vi "Renderizado.vi"() -> ()   [LabVIEW 2016]
uses:
  <vilib>/picture/3D Picture Control/Object/Create Object (drawable).vi
  <vilib>/picture/3D Picture Control/Helpers/Apply Texture (no reference).vi
  <vilib>/picture/3D Picture Control/NI_3D Picture Control.lvlib
panel:
  in  "angle":sgl(knob) scale=0.0..180.0
  in  "Stop Button":bool
  in  "Path":path
  in  "Enum":enum16{"Esfera", "Cubo", "Cilindro", "Cono"}(ring)
  out "3D Picture":refnum<vi>(3d-picture)
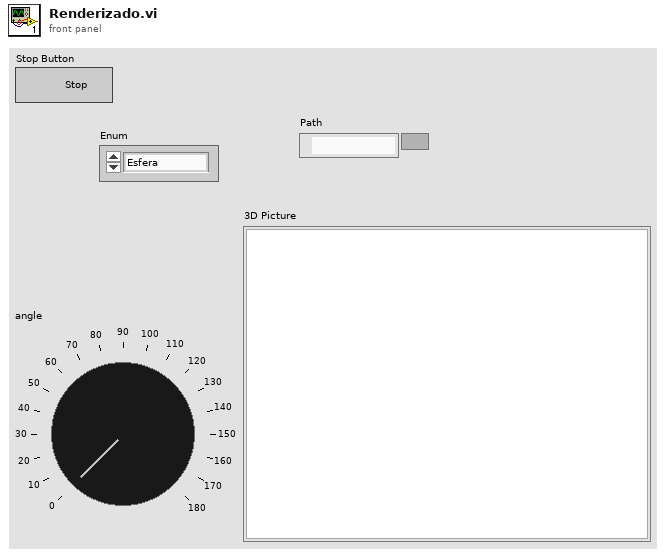
[diagram p1: front panel]
types:
  T1 = cluster{"Red":sgl, "Green":sgl, "Blue":sgl, "Alpha":sgl}
  T2 = typedef "imagedata.ctl" = cluster{"image type":i32, "image depth":i32, "image":u8[], "mask":u8[], "colors":u32[], "Rectangle":cluster{"left":i16, "top":i16, "right":i16, "bottom":i16}}
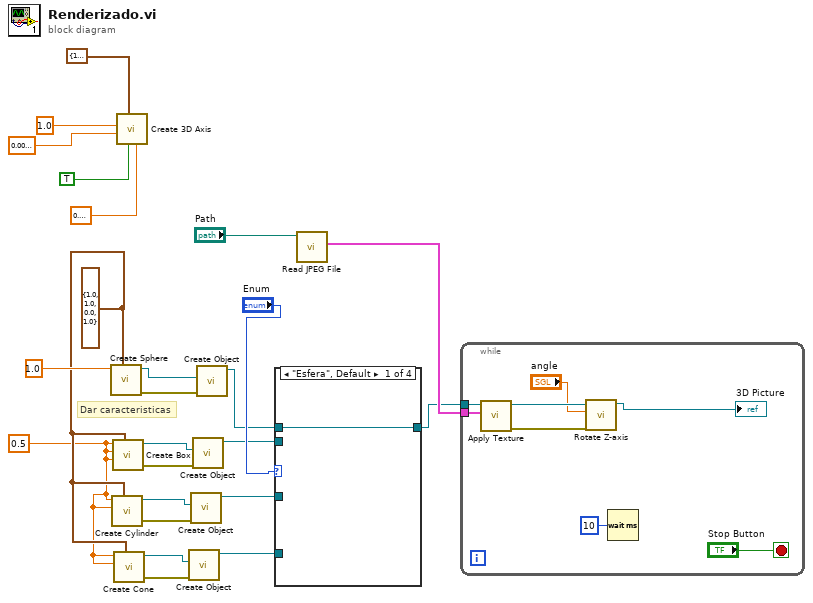
[diagram p0: block diagram]
diagram:
  w9 = sgl 0.5 ("Length X")
  w16 = T1 {"Red"=1.0, "Green"=1.0, "Blue"=0.0, "Alpha"=1.0} ("Color")
  # "Dar caracteristicas"
  n1 = call <vilib>:"Create Sphere.vi"("Color"=w16, "Radius"=sgl 1.0) -> ("error out"=w18:errorcluster, "New Sphere Refnum"=w17:refnum<vi>)  [unwired: 8 in]
  n2 = call <vilib>:"Create Cylinder.vi"("Color"=w16, "Radius"=w9, "Height"=w9) -> ("error out"=w13:errorcluster, "New Cylinder Refnum"=w12:refnum<vi>)  [unwired: 7 in]
  n3 = call <vilib>:"Create Box.vi"("Color"=w16, "Length Z"=w9, "Length Y"=w9, "Length X"=w9) -> ("error out"=w11:errorcluster, "New Box Refnum"=w10:refnum<vi>)  [unwired: 6 in]
  n4 = call <vilib>:"Create Cone.vi"("Color"=w16, "Radius"=w9, "Height"=w9) -> ("error out"=w15:errorcluster, "New Cone Refnum"=w14:refnum<vi>)  [unwired: 7 in]
  n5 = call <vilib>:"Create 3D Axis.vi"("Character Size"=sgl 0.1, "Axis label?"=TRUE, "Color"=T1 {"Red"=1.0, "Green"=0.0, "Blue"=0.0, "Alpha"=1.0}, "Radius"=sgl 0.01, "Length"=sgl 1.0) -> ()  [unwired: 5 in, 2 out]
  n6 = call-poly <vilib>:"Create Object.vi"("error in (no error)"=w15, "Geometry"=w14) -> ("Scene:New Object"=w4:refnum<vi>)  [unwired: 8 in, 1 out]
  n7 = call-poly <vilib>:"Create Object.vi"("error in (no error)"=w13, "Geometry"=w12) -> ("Scene:New Object"=w5:refnum<vi>)  [unwired: 8 in, 1 out]
  n8 = call-poly <vilib>:"Create Object.vi"("error in (no error)"=w11, "Geometry"=w10) -> ("Scene:New Object"=w6:refnum<vi>)  [unwired: 8 in, 1 out]
  n9 = call-poly <vilib>:"Create Object.vi"("error in (no error)"=w18, "Geometry"=w17) -> ("Scene:New Object"=w7:refnum<vi>)  [unwired: 8 in, 1 out]
  n10 = case shown="\"Esfera\", Default" "Enum" {
    tunnel: w7 -> [w25 _ _ _]
    tunnel: [w25 w26 w27 w28] -> w1
    tunnel: w6 -> [_ w26 _ _]
    tunnel: w5 -> [_ _ w27 _]
    tunnel: w4 -> [_ _ _ w28]
    frame "Esfera", Default {
    }
    frame "Cubo" {
    }
    frame "Cilindro" {
    }
    frame "Cono" {
    }
  }
  n11 = call <vilib>:"Read JPEG File.vi"("path to JPEG file"="Path") -> ("image data"=w2:T2)  [unwired: 8 in, 2 out]
  n12 = while {
    tunnel: w2 -> [w36]
    tunnel: w1 -> [w35]
    stop <- "Stop Button" stop-if-true
    n13 = call-poly <vilib>:"Apply Texture.vi"("Image Data"=w36, "Scene Object In"=w35) -> ("error out"=w31:errorcluster, "Scene Object Out"=w32:refnum<vi>)  [unwired: 8 in]
    n14 = call <vilib>:"Rotate Z-axis.vi"("error in (no error)"=w31, "angle"="angle", "Scene Object In"=w32) -> ("Scene Object Out"=→"3D Picture":refnum<vi>)  [unwired: 7 in, 1 out]
    n15 = Wait (ms)(milliseconds to wait=u32 10) -> ()  [unwired: 1 out]
  }
